vi "Mcp2210 Get Gpio Pin Val.vi"(8 "error in (no error)":errorcluster, 11 "handle":i32) -> (0 "error out":errorcluster, 2 "GPIO Output":bool[](array[boolean]), 3 "handle out":i32)   [LabVIEW 2015, in "mcp2210.lvlib"]
doc: "Provides the current GPIO values. The values are valid only for the pins\npreviously configured as GPIOs.\nParameters:\nInputs:\n- void *handle - The pointer to the device handle. Cannot be NULL.\nOutputs:\n- unsigned int *pgpioPinVal - GPIO pin values, if successful call. In case of error the value\nis not changed.\nCannot be NULL pointer.\nReturns:\n- 0 for success: E_SUCCESS\n- negative error code: E_ERR_NULL, E_ERR_INVALID_HANDLE_VALUE\nE_ERR_UNKOWN_ERROR, E_ERR_INVALID_PARAMETER\nE_ERR_HID_TIMEOUT, E_ERR_HID_RW_FILEIO\nE_ERR_CMD_ECHO, E_ERR_CMD_FAILED\n\nMCP2210_DLL_UM_API int __stdcall Mcp2210_GetGpioPinVal(void *handle, unsigned int *pgpioPinVal);"
uses:
  <userlib>/mcp2210/mcp2210.lvlib
  <userlib>/mcp2210/mcp2210_dll_um_x86.dll
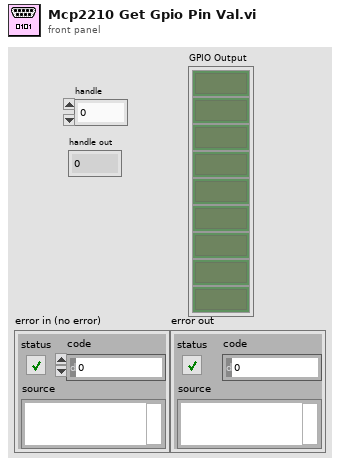
[diagram p1: front panel]
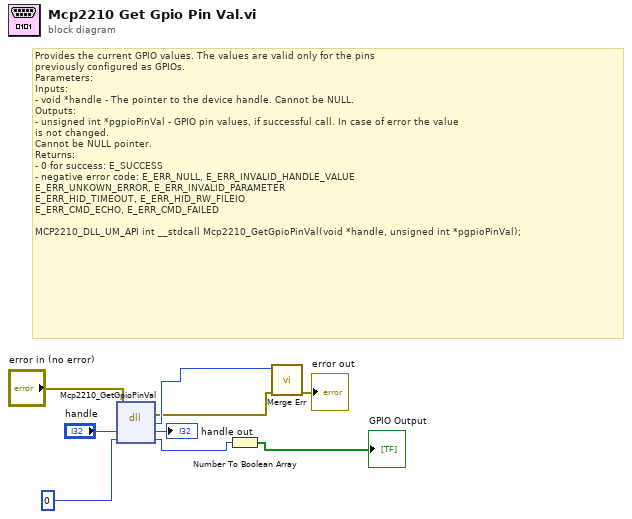
[diagram p0: block diagram]
diagram:
  # "Provides the current GPIO values. The values are valid only for the pins\npreviously configured as GPIOs.\nParameters:\nInputs:\n- void *handle - The pointer to the device handle. Cannot be NULL.\nOutputs:\n- unsigned int *pgpioPinVal - GPIO pin values, if successful call. In case of error the value\nis not changed.\nCannot be NULL pointer.\nReturns:\n- 0 for success: E_SUCCESS\n- negative error code: E_ERR_NULL, E_ERR_INVALID_HANDLE_VALUE\nE_ERR_UNKOWN_ERROR, E_ERR_INVALID_PARAMETER\nE_ERR_HID_TIMEOUT, E_ERR_HID_RW_FILEIO\nE_ERR_CMD_ECHO, E_ERR_CMD_FAILED\n\nMCP2210_DLL_UM_API int __stdcall Mcp2210_GetGpioPinVal(void *handle, unsigned int *pgpioPinVal);"
  n1 = dll-call lib="D:/LabVIEW 2015/user.lib/mcp2210/mcp2210_dll_um_x86.*" fn="Mcp2210_GetGpioPinVal"(error in="error in (no error)", "handle"="handle", "pgpioPinVal"=u32 0) -> (error out=w5:errorcluster, "return type"=w6:i32, "handle"=→"handle out":i32, "pgpioPinVal"=w2:u32)  [unwired: 2 in, 1 out]
  n2 = Number To Boolean Array(number=w2) -> (Boolean array=→"GPIO Output":bool[])
  n3 = call <userlib>:"Merge Err.vi"("error in (no error)"=w5, "return type"=w6) -> ("error out"=→"error out":errorcluster)  [unwired: 9 in]
